vi "GetSectionData.vi"(7 "SectionName":string, 8 "error in":errorcluster, 11 "ConfigRef":T1) -> (0 "error out":errorcluster, 2 "Data":string[][](array[string]), 3 "ConfigRefOut":T1)   [LabVIEW 2010]
uses:
  <vilib>/Utility/config.llb/Config Data RefNum.ctl
  <vilib>/Utility/config.llb/Read Key (String).vi
  <vilib>/Utility/config.llb/NI_LVConfig.lvlib
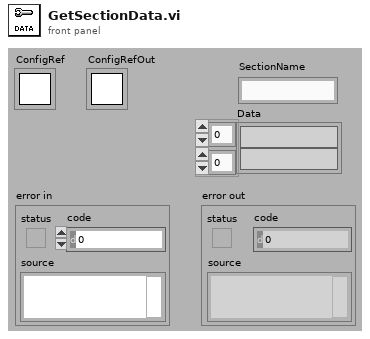
[diagram p1: front panel]
types:
  T1 = typedef "NI_LVConfig.lvlib/Config Data RefNum.ctl" = refnum<k1>
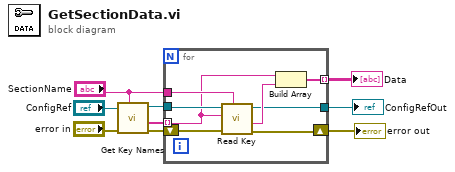
[diagram p0: block diagram]
diagram:
  n1 = call <vilib>:"Get Key Names.vi"("section"="SectionName", "error in (no error)"="error in", "refnum"="ConfigRef") -> ("error out"=w5:errorcluster, "key names"=w3:string[], "refnum out"=w4:T1)  [unwired: 5 in, 1 out]
  n2 = for {
    shift-right: [w12] -> w6
    shift-left: w5 -> [w17]
    tunnel: w4 -> [w16]
    tunnel: w3 -> [w14] mode=indexing
    tunnel: "SectionName" -> [w15]
    tunnel: [w11] -> w2 mode=indexing
    tunnel: [w10] -> w8
    n3 = call-poly <vilib>:"Read Key.vi"("section"=w15, "error in (no error)"=w17, "key"=w14, "refnum"=w16) -> ("error out"=w12:errorcluster, "value"=w13:string, "refnum out"=w10:T1)  [unwired: 4 in, 1 out]
    n4 = Build Array(w14, w13) -> (w11:string[])
  }
  "error out" <- w6
  "ConfigRefOut" <- w8
  "Data" <- w2
